vi "Datos_TestStand.vi"(10 "Arr of Clstr":cluster{"Numeric":dbl, "String":string}[](array[cluster]), 11 "Array":dbl[](array[numeric])) -> (2 "Arr_Clstr_Out":cluster{"Numeric":dbl, "String":string}[](array[cluster]), 3 "Array_out":dbl[](array[numeric]))   [LabVIEW 2024]
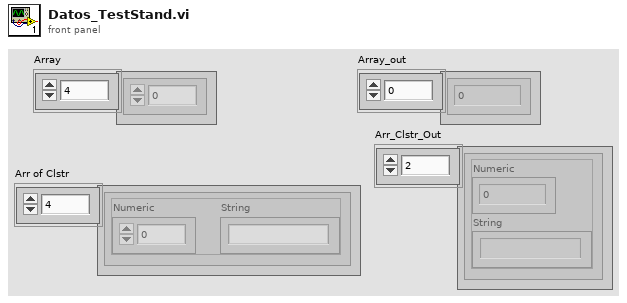
[diagram p1: front panel]
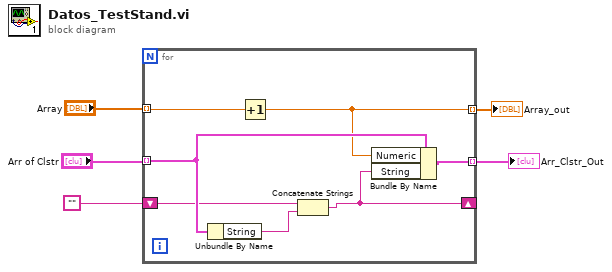
[diagram p0: block diagram]
diagram:
  n1 = for {
    tunnel: "Array" -> [w12] mode=indexing
    tunnel: [w10] -> w4 mode=indexing
    tunnel: "Arr of Clstr" -> [w11] mode=indexing
    tunnel: [w9] -> w2 mode=indexing
    shift-right: [w6] -> _
    shift-left: "" -> [w7]
    n2 = Unbundle By Name(w11) -> ("String"=w8:string)
    n3 = Increment(x=w12) -> (x+1=w10:dbl)
    n4 = Concatenate Strings(w7, w8) -> (w6:string)
    n5 = Bundle By Name(cluster=w11, "Numeric"=w10, "String"=w6) -> (w9:cluster{"Numeric":dbl, "String":string})
  }
  "Array_out" <- w4
  "Arr_Clstr_Out" <- w2
